vi "LoadIon.vi"(11 "Threshold":u32) -> (3 "Ion":bool)   [LabVIEW 2009]
uses:
  <vilib>/DAQmx/configure/timing.llb/DAQmx Timing (Sample Clock).vi
  <vilib>/DAQmx/create/channels.llb/DAQmx Create Channel (CI-Count Edges).vi
  <vilib>/DAQmx/read.llb/DAQmx Read (Counter U32 1Chan 1Samp).vi
  Program Files/National Instruments/LabVIEW 2009/resource/objmgr/daqmx.rc
  <vilib>/Analysis/NI_AALBase.lvlib
panel:
  out "Counts":u32
  out "Mean/Variance":dbl
  out "Variance":dbl format="%0.2f"
  out "Mean":dbl format="%0.2f"
  in  "Sample rate":dbl=50.0 format="%0.2f"
  in  "Samples per averaging\nblock":i32=100 min=1 step=1
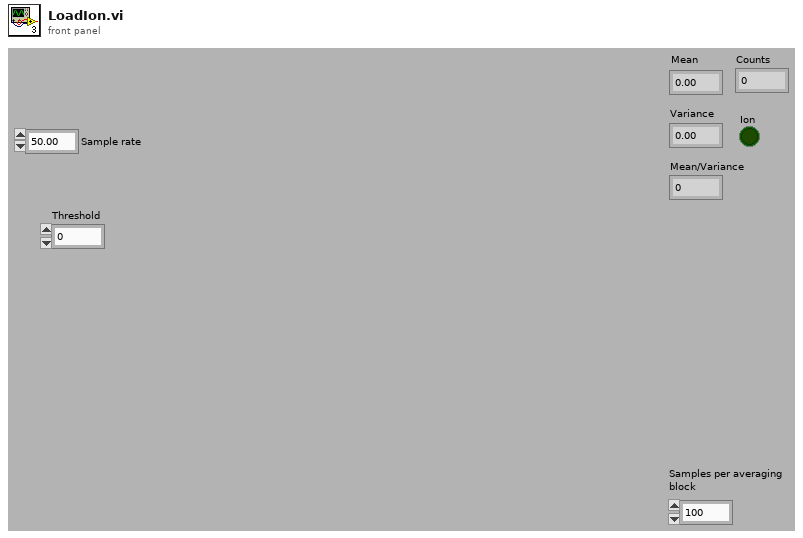
[diagram p1: front panel]
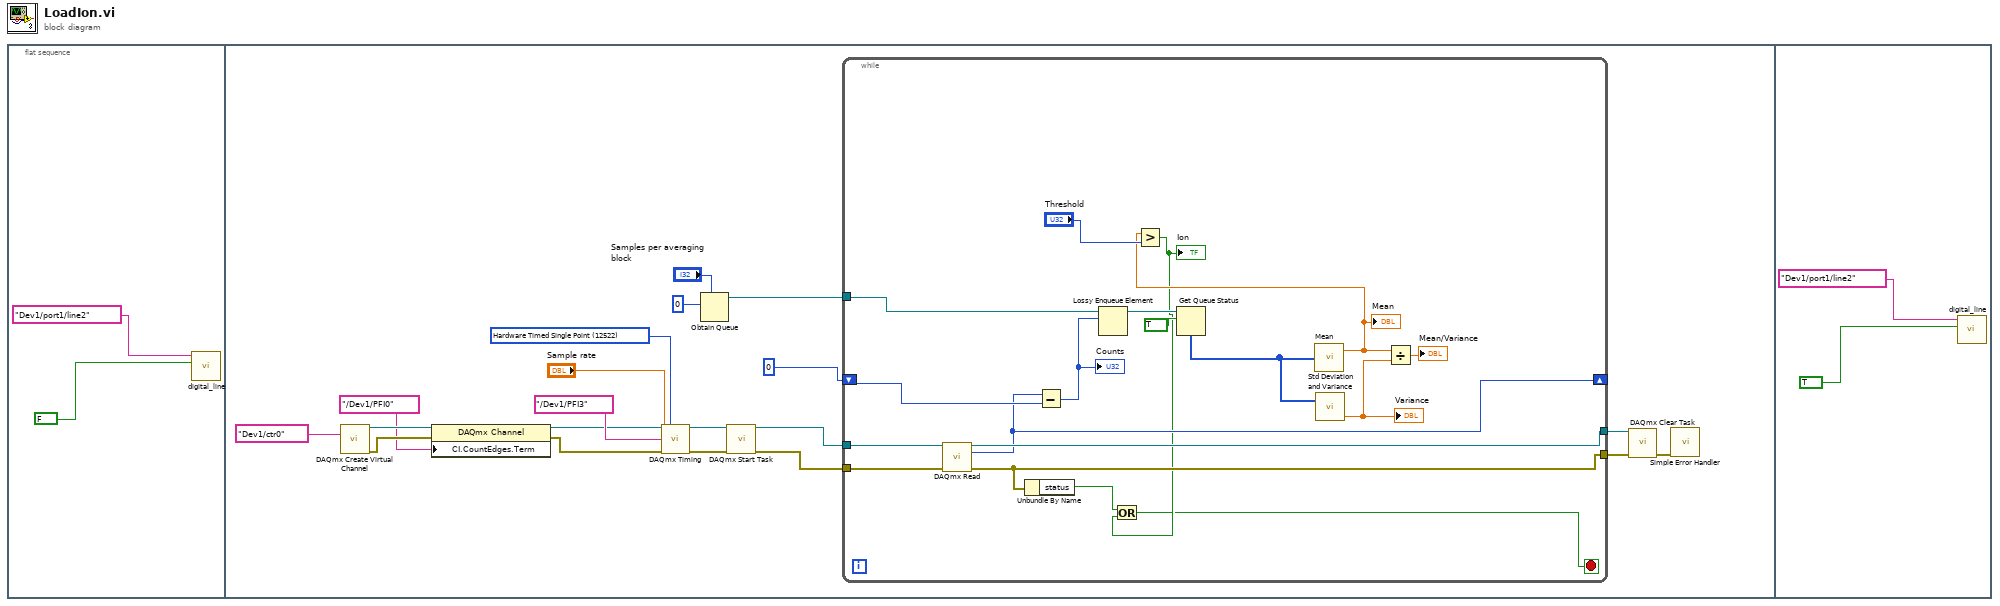
[diagram p0: block diagram]
diagram:
  n1 = flat-sequence {
    frame #0 {
      n2 = call "digital_line.vi"("NewVal"=FALSE, "lines"=tag "Dev1/port1/line2") -> ()  [unwired: 2 in]
    }
    frame #1 {
      w10 = 12522 items=["Finite Samples"=10178, "Continuous Samples"=10123, "Hardware Timed Single Point"=12522] ("sample mode")
      n3 = call-poly <vilib>:"DAQmx Create Virtual Channel.vi"("counter"=tag "Dev1/ctr0") -> ("task out"=w16:refnum<k21>, "error out"=w15:errorcluster)  [unwired: 13 in]
      n4 = property class="DAQmx Channel"(reference=w16, error in=w15, "CI.CountEdges.Term"=tag "/Dev1/PFI0") -> (reference out=w18:refnum<k21>, error out=w17:errorcluster)
      n5 = call-poly <vilib>:"DAQmx Timing.vi"("task/channels in"=w18, "sample mode"=w10, "rate"="Sample rate", "source"=tag "/Dev1/PFI3", "error in"=w17) -> ("task out"=w21:refnum<k21>, "error out"=w20:errorcluster)  [unwired: 9 in]
      n6 = Obtain Queue(max queue size (-1, unlimited)="Samples per averaging\nblock", element data type=u32 0) -> (queue out=w9:refnum<queue>)  [unwired: 3 in, 2 out]
      n7 = call <vilib>:"DAQmx Start Task.vi"("task/channels in"=w21, "error in"=w20) -> ("task out"=w7:refnum<k21>, "error out"=w6:errorcluster)  [unwired: 12 in]
      n8 = while {
        tunnel: w9 -> [w31]
        shift-right: [w25] -> _
        shift-left: u32 0 -> [w30]
        tunnel: w7 -> [w29]
        tunnel: w6 -> [w28]
        tunnel: [w27] -> w4
        tunnel: [w26] -> w3
        stop <- w23 stop-if-true
        n9 = call-poly <vilib>:"DAQmx Read.vi"("task/channels in"=w29, "error in"=w28) -> ("task out"=w27:refnum<k21>, "data"=w25:u32, "error out"=w26:errorcluster)  [unwired: 11 in]
        n10 = Unbundle By Name(w26) -> ("status"=w40:bool)
        n11 = Subtract(x=w25, y=w30) -> (x-y=w33:u32)
        "Counts" <- w33
        n12 = Lossy Enqueue Element(queue=w31, element=w33) -> (queue out=w39:refnum<queue>)  [unwired: 1 in, 3 out]
        n13 = Get Queue Status(queue=w39, return elements? (F)=TRUE) -> (elements=w34:u32[])  [unwired: 1 in, 7 out]
        n14 = call <vilib>:"Mean.vi"("X"=w34) -> ("mean"=w32:dbl)  [unwired: 1 out]
        "Mean" <- w32
        n15 = Greater?(x=w32, y="Threshold") -> (0:w24:bool)
        "Ion" <- w24
        n16 = Or(x=w40, y=w24) -> (x .or. y?=w23:bool)
        n17 = call <vilib>:"Std Deviation and Variance.vi"("X"=w34) -> ("variance"=w37:dbl)  [unwired: 1 in, 2 out]
        "Variance" <- w37
        n18 = Divide(x=w32, y=w37) -> (x/y=→"Mean/Variance":dbl)
      }
      n19 = call <vilib>:"DAQmx Clear Task.vi"("task in"=w4, "error in"=w3) -> ("error out"=w5:errorcluster)  [unwired: 13 in]
      n20 = call <vilib>:"Simple Error Handler.vi"("error in (no error)"=w5) -> ()  [unwired: 4 in, 5 out]
    }
    frame #2 {
      n21 = call "digital_line.vi"("NewVal"=TRUE, "lines"=tag "Dev1/port1/line2") -> ()  [unwired: 2 in]
    }
  }
